vi "Abort All.vi"(8 "error in (no error)":errorcluster) -> (0 "error out":errorcluster)   [LabVIEW 2020, in "Architecture Support.lvlib"]
uses:
  Architecture Support.lvlib
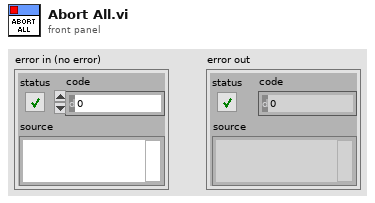
[diagram p1: front panel]
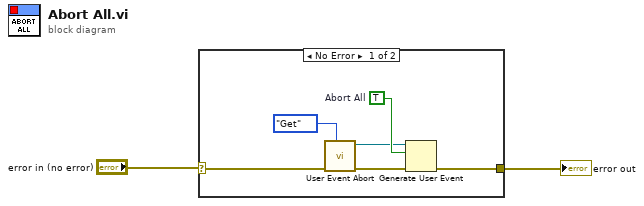
[diagram p0: block diagram]
diagram:
  n1 = case shown="No Error" "error in (no error)" {
    selector: "error in (no error)" -> [w8 w9]
    tunnel: [w4 w9] -> w1
    frame No Error {
      w6 = TRUE  # Abort All
      n2 = call "User Event Abort.vi"("Enum"=enum16{"Create", "Destroy", "Get"}."Get", "error in (no error)"=w8) -> ("error out"=w5:errorcluster, "User Event Out"=w3:refnum<user-event>)  [unwired: 8 in]
      n3 = Generate User Event(user event=w3, event data cluster=w6, error in=w5) -> (error out=w4:errorcluster)  [unwired: 1 in, 1 out]
    }
    frame Error {
    }
  }
  "error out" <- w1
